vi "RegisterAppender.vi"(8 "error in (no error)":errorcluster, 10 "Lumberjack.lvlib:Appender.lvclass":refnum<class "Appender.lvclass">, 11 "Logger in":refnum<class "Logger.lvclass">) -> (0 "error out":errorcluster, 3 "Logger out":refnum<class "Logger.lvclass">)   [LabVIEW 2026, in "Lumberjack.lvlib" / "Logger.lvclass"]
doc: "Registers a constructed, configured appender with the running logger and blocks until it is live. Sends RegisterAppenderMsg to the LogManager (which launches the appender as a nested actor and posts an updated Snapshot), then blocks on WaitForSnapshot(IDPresent, id) until the appender's id appears in a Snapshot, so the next Log reaches it (SRS-LMBR-020, 028). The id is read from the appender's common config (GetID). No-op passthrough if no logger resolves (+29). Control plane; not on the hot path."
uses:
  Logger.lvclass
  Core/Appenders/Appender.lvclass/Appender.lvclass
  Logger.lvclass/Logger.ctl
  TypeDefs/SnapshotWaitMode.ctl
  <vilib>/ActorFramework/Message Enqueuer/Message Enqueuer.lvclass
  Core/Messages/RegisterAppenderMsg.lvclass/RegisterAppenderMsg.lvclass
  Lumberjack.lvlib
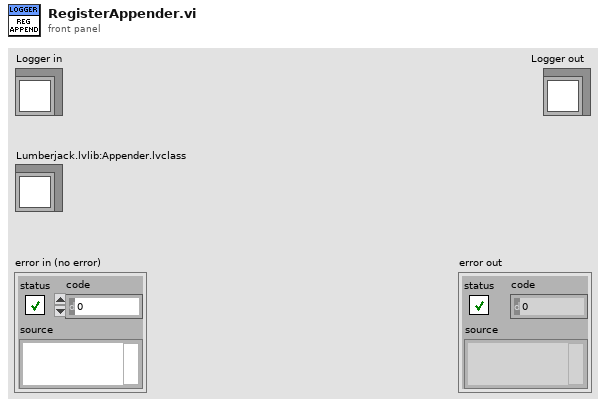
[diagram p1: front panel]
types:
  T1 = typedef "Lumberjack.lvlib/SnapshotWaitMode.ctl" = enum16{"AnySnapshot", "IDPresent", "IDAbsent"}
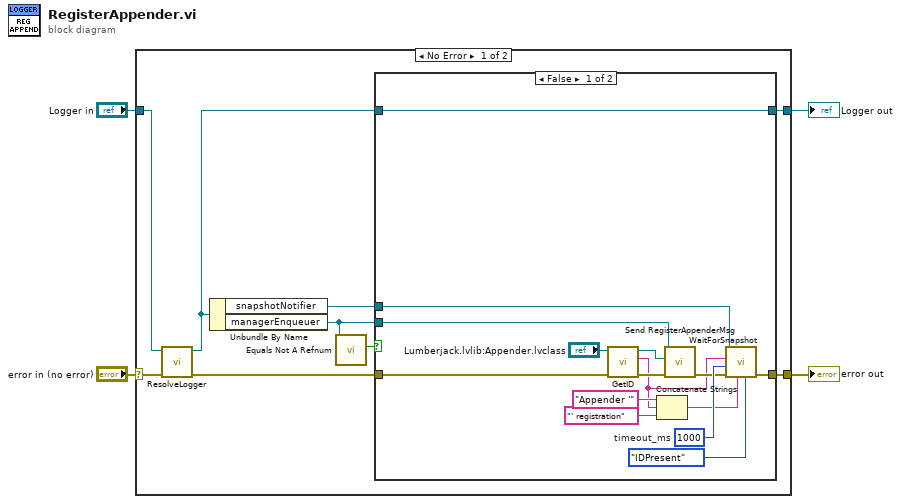
[diagram p0: block diagram]
diagram:
  n1 = case shown="No Error" "error in (no error)" {
    selector: "error in (no error)" -> [w13 w32]
    tunnel: [w7 w32] -> w3
    tunnel: [w11 w31] -> w1
    tunnel: "Logger in" -> [w12 w31]
    frame No Error {
      n2 = call "ResolveLogger.vi"("error in (no error)"=w13, "Logger in"=w12) -> ("error out"=w6:errorcluster, "Logger out"=w10:refnum<class "Logger.lvclass">)  [unwired: 8 in]
      n3 = Unbundle By Name(w10) -> ("snapshotNotifier"=w5:refnum<notifier>, "managerEnqueuer"=w8:refnum<class "Message Enqueuer.lvclass">)
      n4 = call <vilib>:"Equals Not A Refnum.vi"("Message Enqueuer"=w8) -> ("Not a refnum?"=w9:bool)  [unwired: 10 in]
      n5 = case shown="False" w9 {
        tunnel: w6 -> [w22 w29]
        tunnel: [w28 w30] -> w11
        tunnel: w10 -> [w28 w30]
        tunnel: w8 -> [w27 _]
        tunnel: w5 -> [w25 _]
        tunnel: [w26 w29] -> w7
        frame False {
          w24 = 1000  # timeout_ms
          n6 = call "GetID.vi"("error in (no error)"=w22, "Appender in"="Lumberjack.lvlib:Appender.lvclass") -> ("error out"=w20:errorcluster, "ID"=w14:string, "Appender out"=w21:refnum<class "Appender.lvclass">)  [unwired: 7 in]
          n7 = Concatenate Strings("Appender '" ("Context"), w14, "' registration" ("Context")) -> (w16:string)
          n8 = call "Send RegisterAppenderMsg.vi"("error in (no error)"=w20, "Lumberjack.lvlib:Appender.lvclass"=w21, "Enqueuer in"=w27) -> ("error out"=w19:errorcluster)  [unwired: 7 in, 1 out]
          n9 = call "WaitForSnapshot.vi"("SnapshotWaitMode"=SnapshotWaitMode."IDPresent", "Context"=w16, "error in (no error)"=w19, "timeout_ms"=w24, "targetID"=w14, "notifier"=w25) -> ("error out"=w26:errorcluster)  [unwired: 4 in, 1 out]
        }
        frame True {
        }
      }
    }
    frame Error {
    }
  }
  "error out" <- w3
  "Logger out" <- w1
